vi "RenderGeometry.vi"(7 "Texture [SDL_Texture *] (NULL)":i64 format="%.0x", 8 "No Error":errorcluster, 9 "Indices (Empty)":i32[](array[numeric]), 10 "Vertices":T1[](array[typedef]), 11 "Renderer [SDL_Renderer *]":i64 format="%.0x") -> (0 "error out":errorcluster)   [LabVIEW 2024, in "SDL3.lvlib" / "Render.lvlib"]
doc: "<B>Summary</B>\nRender a list of triangles, optionally using a texture and indices into the vertex array Color and alpha modulation is done per vertex (<B>SDL_SetTextureColorMod</B> and <B>SDL_SetTextureAlphaMod</B> are ignored)."
uses:
  Render.lvlib
  Lib/SDL3.dll
  Rect/FPoint--cluster.ctl
  Pixels/FColor--cluster.ctl
  Vertex--cluster.ctl
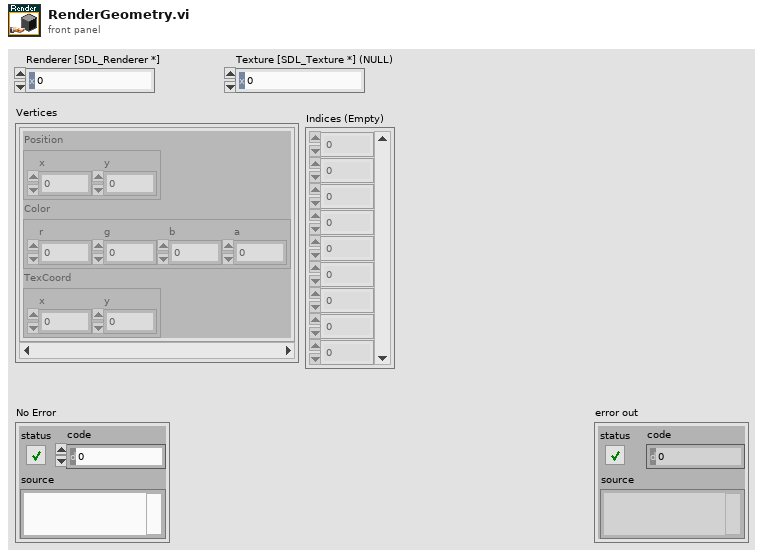
[diagram p1: front panel]
types:
  T1 = typedef "SDL3.lvlib/Render.lvlib/Vertex--cluster.ctl" = cluster{"Position":T2, "Color":T3, "TexCoord":T2}
  T2 = typedef "SDL3.lvlib/Rect.lvlib/FPoint--cluster.ctl" = cluster{"x":sgl, "y":sgl}
  T3 = typedef "SDL3.lvlib/Pixels.lvlib/FColor--cluster.ctl" = cluster{"r":sgl, "g":sgl, "b":sgl, "a":sgl}
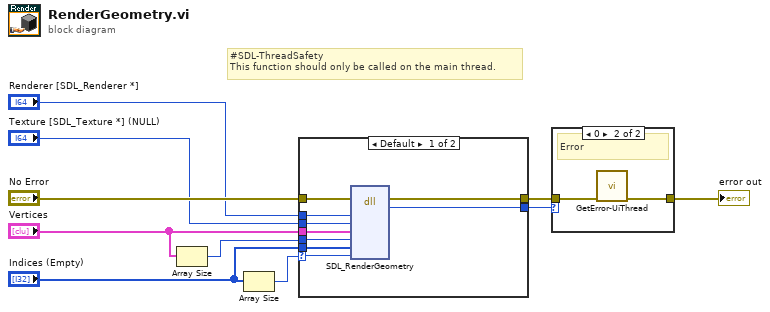
[diagram p0: block diagram]
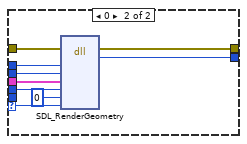
[diagram p2: hidden frame]
diagram:
  # "#SDL-ThreadSafety\nThis function should only be called on the main thread."
  n1 = Array Size(array="Vertices") -> (size(s)=w4:i32)
  n2 = Array Size(array="Indices (Empty)") -> (size(s)=w1:i32)
  n3 = case shown="Default" w1 {
    selector: w1 -> [w11 w21]
    tunnel: "No Error" -> [w19 w28]
    tunnel: "Renderer [SDL_Renderer *]" -> [w18 w27]
    tunnel: "Texture [SDL_Texture *] (NULL)" -> [w17 w26]
    tunnel: [w16 w25] -> w6
    tunnel: [w15 w24] -> w5
    tunnel: w4 -> [w14 w23]
    tunnel: "Vertices" -> [w13 w22]
    tunnel: "Indices (Empty)" -> [w12 _]
    frame Default {
      n4 = dll-call lib="C:/Users/Thomas/Documents/Projects/LV-SDL3/Sources/SDL3/Lib/SDL3.*" fn="SDL_RenderGeometry"(error in=w19, "renderer"=w18, "texture"=w17, "vertices"=w13, "num_vertices"=w14, "indices"=w12, "num_indices"=w11) -> (error out=w16:errorcluster, "return type"=w15:i32)  [unwired: 8 in, 1 out]
    }
    frame 0 {
      n5 = dll-call lib="C:/Users/Thomas/Documents/Projects/LV-SDL3/Sources/SDL3/Lib/SDL3.*" fn="SDL_RenderGeometry"(error in=w28, "renderer"=w27, "texture"=w26, "vertices"=w22, "num_vertices"=w23, "indices"=i64 0, "num_indices"=w21) -> (error out=w25:errorcluster, "return type"=w24:i32)  [unwired: 8 in, 1 out]
    }
  }
  n6 = case shown="0" w5 {
    tunnel: w6 -> [w29 w31]
    tunnel: [w29 w30] -> w9
    frame Default {
      # "Ok"
    }
    frame 0 {
      # "Error"
      n7 = call "GetError-UiThread.vi"("No Error"=w31) -> ("error out"=w30:errorcluster)  [unwired: 10 in]
    }
  }
  "error out" <- w9
